vi "无损图层图像匹配3.vi"() -> ()   [LabVIEW 2018]
uses:
  <vilib>/vision/NI_Vision_Development_Module.lvlib
panel:
  out "Matches (real-world)":T1(array[cluster]) {"Bounding Box"."y" format="%.2f"; "Bounding Box"."x" format="%.2f"; "Score" format="%.2f"; "Scale" format="%.2f"; "Angle" format="%.2f"; "Position"."y" format="%.2f"; "Position"."x" format="%.2f"}
  out "Image 2":T2(plugin-control)
  out "Number of Matches":i32
  out "error out":errorcluster
  out "Image":T2(plugin-control)
  out "文件名":string[](array[string])
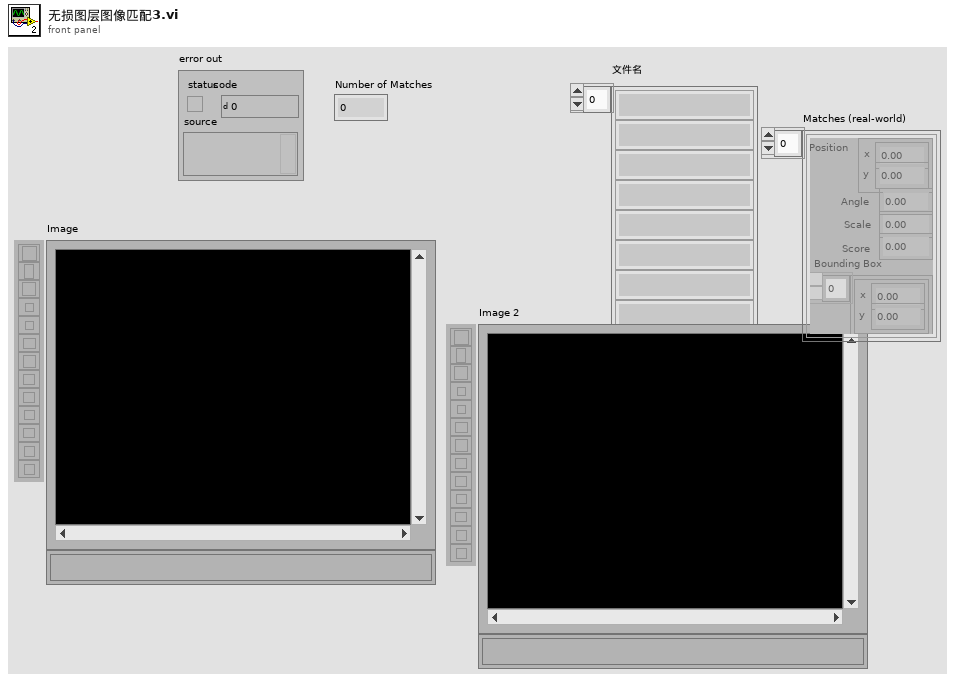
[diagram p1: front panel]
types:
  T1 = cluster{"Position":cluster{"x":sgl, "y":sgl}, "Angle":sgl, "Scale":sgl, "Score":sgl, "Bounding Box":cluster{"x":sgl, "y":sgl}[]}[]
  T2 = typedef "IMAQ Image.ctl" = refnum<image>
  T3 = cluster{"Number of Matches Requested":i32, "Minimum Match Score":sgl, "Angle Ranges":cluster{"Start Angle":sgl, "End Angle":sgl}[]}
  T4 = typedef "Image Type" = u32
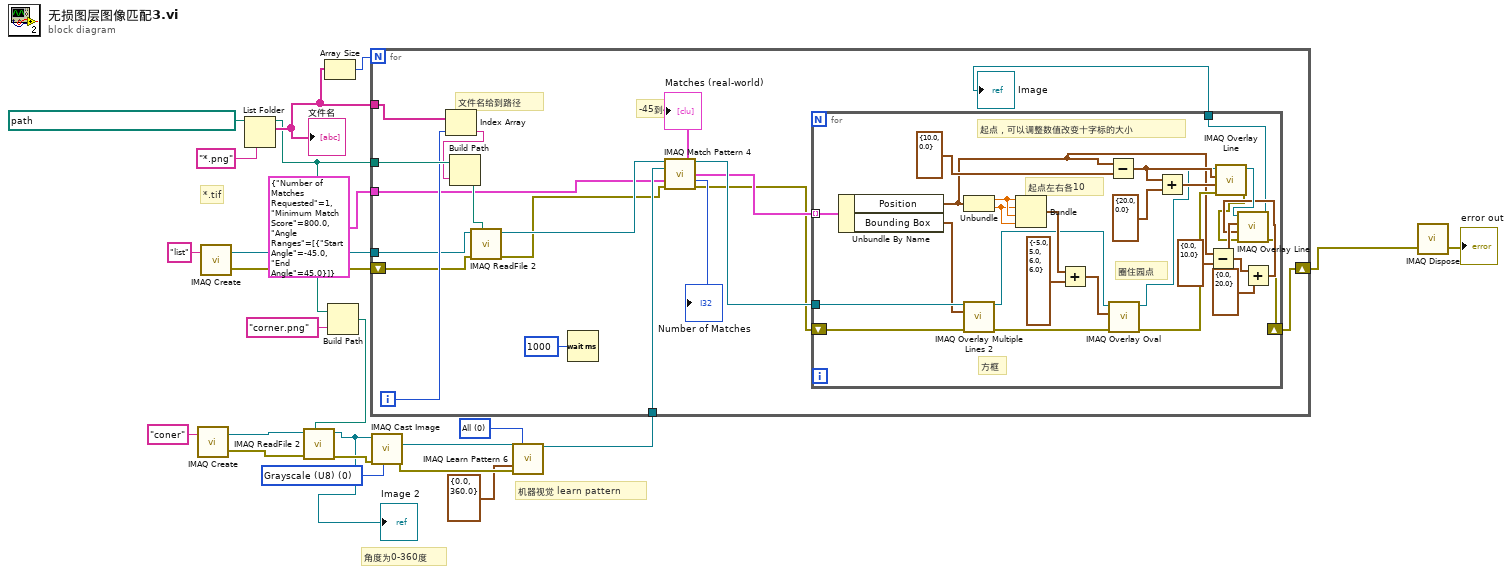
[diagram p0: block diagram]
diagram:
  w5 = 0 items=["All", "Low Discrepancy Sampling", "Grayscale Value Pyramid", "Gradients Pyramid"] ("Algorithm")
  w9 = T4 0 items=["Grayscale (U8)", "Grayscale (I16)", "Grayscale (SGL)", "Complex (CSG)", "RGB (U32)", "HSL (U32)", "RGB (U64)", "Grayscale (U16)"] ("Image Type")
  # "*.tif"
  # "角度为0-360度"
  # "机器视觉 learn pattern"
  n1 = call "IMAQ Create"("Image Name"="coner") -> ("New Image"=w11:T2, "error out"=w10:errorcluster)  [unwired: 4 in]
  n2 = call "IMAQ Create"("Image Name"="list") -> ("New Image"=w22:T2, "error out"=w20:errorcluster)  [unwired: 4 in]
  n3 = List Folder(path=path "D:/Labviewprogram/视觉/Roundcard" ("路径"), pattern="*.png" ("类型")) -> (path out=w15:path, filenames=w17:string[])  [unwired: 2 in, 2 out]
  "文件名" <- w17
  n4 = Array Size(array=w17) -> (size(s)=w16:i32)
  n5 = Build Path(base path=w15, name or relative path="corner.png" ("名称或相对路径")) -> (appended path=w12:path)
  n6 = call "IMAQ ReadFile 2"("File Path"=w12, "error in (no error)"=w10, "Image"=w11) -> ("error out"=w8:errorcluster, "Image Out"=w2:T2)  [unwired: 4 in, 3 out]
  "Image 2" <- w2
  n7 = call "IMAQ Cast Image"("Image Type"=w9, "error in (no error)"=w8, "Image Src"=w2) -> ("error out"=w6:errorcluster, "Image Dst Out"=w7:T2)  [unwired: 7 in]
  n8 = call "IMAQ Learn Pattern 6"("Image"=w7, "Algorithm"=w5, "Angle Range"=cluster{"Start Angle":sgl, "End Angle":sgl} {"Start Angle"=0.0, "End Angle"=360.0}, "error in (no error)"=w6) -> ("Template Image Out"=w3:T2)  [unwired: 9 in, 2 out]
  n9 = for {
    N: w16 -> [_]
    tunnel: w17 -> [w42]
    tunnel: w15 -> [w41]
    tunnel: w22 -> [w38]
    shift-right: [w27] -> w19
    shift-left: w20 -> [w37]
    tunnel: w3 -> [w34]
    tunnel: T3 {"Number of Matches Requested"=1, "Minimum Match Score"=800.0, "Angle Ranges"=[{"Start Angle"=-45.0, "End Angle"=45.0}]} -> [w25]
    i -> [w40]
    # "-45到45度"
    # "文件名给到路径"
    n10 = Index Array(array=w42, index=w40) -> (element=w39:string)
    n11 = Build Path(base path=w41, name or relative path=w39) -> (appended path=w31:path)
    n12 = call "IMAQ ReadFile 2"("File Path"=w31, "error in (no error)"=w37, "Image"=w38) -> ("error out"=w33:errorcluster, "Image Out"=w35:T2)  [unwired: 4 in, 3 out]
    n13 = Wait (ms)(milliseconds to wait=u32 1000 ("等待时间（毫秒）")) -> ()  [unwired: 1 out]
    n14 = call "IMAQ Match Pattern 4"("Image"=w35, "Template Image"=w34, "Parameters"=w25, "error in (no error)"=w33) -> ("Image (duplicate)"=w30:T2, "Matches (real-world)"=w29:T1, "Number of Matches"=→"Number of Matches":i32, "error out"=w28:errorcluster)  [unwired: 7 in, 1 out]
    "Matches (real-world)" <- w29
    n15 = for {
      tunnel: w30 -> [w68]
      tunnel: w29 -> [w67] mode=indexing
      shift-right: [w45] -> w27
      shift-left: w28 -> [w65]
      tunnel: [w43] -> w26
      # "起点左右各10"
      # "起点，可以调整数值改变十字标的大小"
      # "方框"
      # "圈住园点"
      n16 = Unbundle By Name(w67) -> ("Position"=w52:cluster{"x":sgl, "y":sgl}, "Bounding Box"=w66:cluster{"x":sgl, "y":sgl}[])
      n17 = Unbundle(w52) -> ("x"=w64:sgl, "y"=w63:sgl)
      n18 = call "IMAQ Overlay Multiple Lines 2"("Image"=w68, "Line End Points"=w66, "error in (no error)"=w65) -> ("Image Out"=w59:T2, "error out"=w58:errorcluster)  [unwired: 11 in]
      n19 = Bundle("x"=w64, "y"=w63, "x"=w64, "y"=w63) -> (w62:cluster{"x":sgl, "y":sgl, "x":sgl, "y":sgl})  [unwired: 1 in]
      n20 = Add(x=w62, y=cluster{"x":sgl, "y":sgl, "x":sgl, "y":sgl} {"x"=-5.0, "y"=5.0, "x"=6.0, "y"=6.0}) -> (x+y=w60:cluster{"x":sgl, "y":sgl, "x":sgl, "y":sgl})
      n21 = Subtract(x=w52, y=cluster{"x":sgl, "y":sgl} {"x"=10.0, "y"=0.0}) -> (x-y=w56:cluster{"x":sgl, "y":sgl})
      n22 = call "IMAQ Overlay Oval"("error in (no error)"=w58, "Bounding Rectangle"=w60, "Image"=w59) -> ("error out"=w53:errorcluster, "Image Out"=w44:T2)  [unwired: 7 in]
      n23 = Add(x=w56, y=cluster{"x":sgl, "y":sgl} {"x"=20.0, "y"=0.0}) -> (x+y=w54:cluster{"x":sgl, "y":sgl})
      n24 = Subtract(x=w52, y=cluster{"x":sgl, "y":sgl} {"x"=0.0, "y"=10.0}) -> (x-y=w49:cluster{"x":sgl, "y":sgl})
      n25 = call "IMAQ Overlay Line"("error in (no error)"=w53, "End Point"=w54, "Start Point"=w56, "Image"=w44) -> ("error out"=w46:errorcluster, "Image Out"=w50:T2)  [unwired: 6 in]
      n26 = Add(x=w49, y=cluster{"x":sgl, "y":sgl} {"x"=0.0, "y"=20.0}) -> (x+y=w47:cluster{"x":sgl, "y":sgl})
      n27 = call "IMAQ Overlay Line"("error in (no error)"=w46, "End Point"=w47, "Start Point"=w49, "Image"=w50) -> ("error out"=w45:errorcluster, "Image Out"=w43:T2)  [unwired: 6 in]
    }
    "Image" <- w26
  }
  n28 = call "IMAQ Dispose"("error in (no error)"=w19) -> ("error out"=→"error out":errorcluster)  [unwired: 5 in]
